vi "Autonomous Independent.vi"() -> ()   [LabVIEW 2014]
doc: "This VI is called when autonomous begins, and will automatically be terminated when autonomous ends. You can carry out timed or sensor driven robot movement independently without needing to return to the caller."
uses:
  <vilib>/Rock Robotics/WPI/RobotDrive/WPI_RobotDriveGetSetRefNum.vi
  <vilib>/Rock Robotics/Network Tables/SD Read Number.vi
  <vilib>/Utility/file.llb/Read From Spreadsheet File (DBL).vi
  <vilib>/Rock Robotics/WPI/RobotDrive/WPI_RobotDriveMecanumDrive_Cartesian.vi
  Robot Global Data.vi
panel:
  out "Autonomous Mode to run":T1(ring)
  in  "Ruin from Autonomous VI":bool
  out "Current State":string
  in  "Array":dbl[][](array[numeric])=[[0.0, 2.0], [3.0, 0.0], [0.0, 0.0], [0.0, 0.0]]
  # "[Drive]            [Rotate]             [Lift]                [ Strafe]              [Wait]"
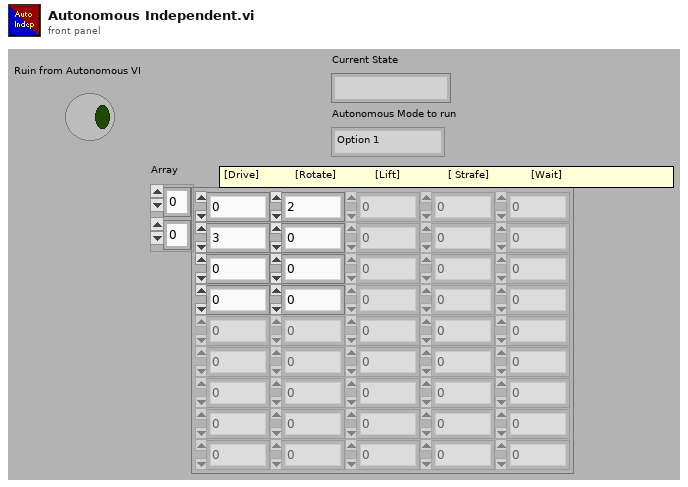
[diagram p1: front panel]
types:
  T1 = enum16{"Option 1", "Option 2", "Option 3", "Option 4", "Option 5", "Option 6"}
  T2 = typedef "WPI_RobotDriveDevRef.ctl" = cluster{"DevStatus":errorcluster, "Motors[]":T3[], "Square Inputs":bool, "Max Output":dbl}
  T3 = typedef "WPI_MotorControlDeviceRef.ctl" = cluster{"DeviceStatus":errorcluster, "Type":T4, "PWM":cluster{"Controller":T5, "PWM Channel":T6, "DeadBand":T7}, "CAN":cluster{"Device Number":u8, "Control Mode":T8, "Semaphore":T9, "Max Vout":dbl, "TalonSRX Control Mode":T10}, "Invert":bool, "TransformRef":T11, "InvTransformRef":T11}
  T4 = typedef "WPI_MotorControlType.ctl" = enum16{"PWM", "CAN", "CANTalonSRX"}
  T5 = typedef "FPGA_TypedefDigitalModule.ctl" = enum16{"Controller 1"}
  T6 = typedef "FPGA_DIOPWMChannel.ctl" = enum8{"PWM 0", "PWM 1", "PWM 2", "PWM 3", "PWM 4", "PWM 5", "PWM 6", "PWM 7", "PWM 8", "PWM 9", "PWM MXP 0", "PWM MXP 1", "PWM MXP 2", "PWM MXP 3", "PWM MXP 4", "PWM MXP 5", "PWM MXP 6", "PWM MXP 7", "PWM MXP 8", "PWM MXP 9", "Invalid"}
  T7 = typedef "WPI_PWMDeadband.ctl" = cluster{"Name":string, "maxPositivePwm":i32, "minPositivePwm":i32, "centerPwm":i32, "maxNegativePwm":i32, "minNegativePwm":i32, "angularRange":u16}
  T8 = typedef "WPI_CANJaguar_ControlMode.ctl" = enum8{"Percent VBus", "Current", "Speed", "Position", "Voltage"}
  T9 = typedef "Semaphore RefNum" = refnum<k1>
  T10 = typedef "WPI_CANTalonSRX_APIControlMode.ctl" = enum8{"Percent VBus", "Speed", "Position", "Slave", "Unchanged / Invalid"}
  T11 = typedef "WPI_PWMTransform_ConPane.ctl" = refnum<vi>
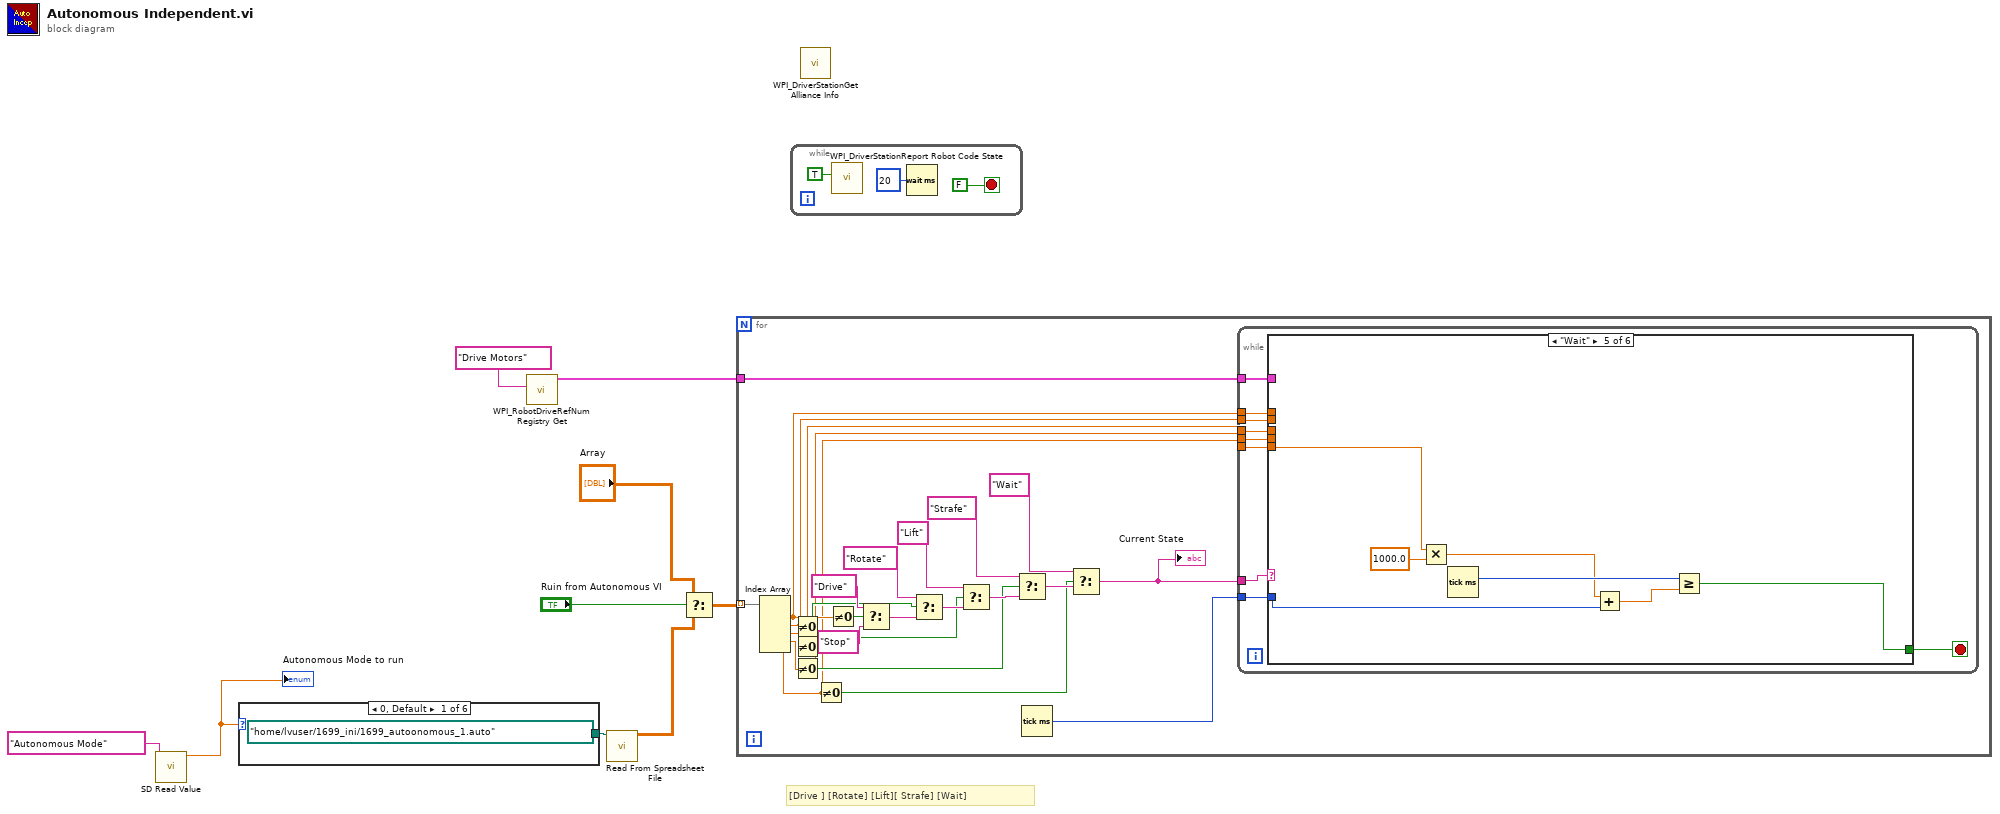
[diagram p0: block diagram]
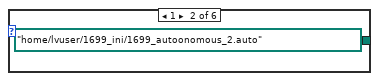
[diagram p2: hidden frame]
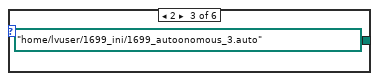
[diagram p3: hidden frame]
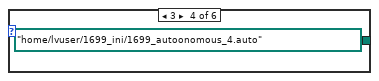
[diagram p4: hidden frame]
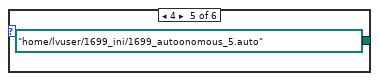
[diagram p5: hidden frame]
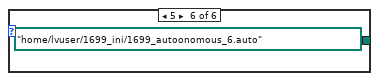
[diagram p6: hidden frame]
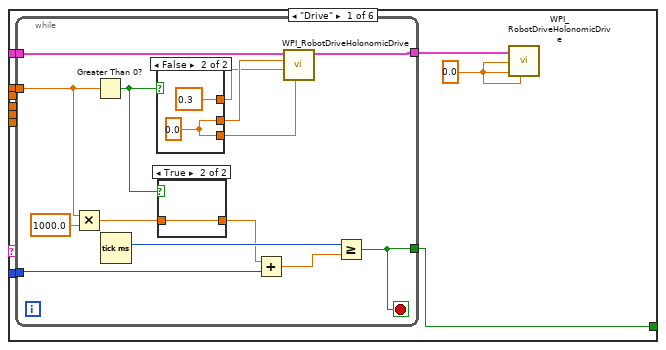
[diagram p7: hidden frame]
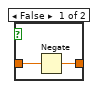
[diagram p8: hidden frame]
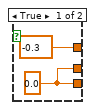
[diagram p9: hidden frame]
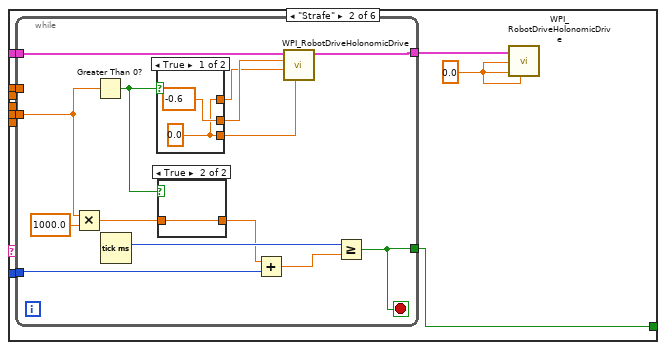
[diagram p10: hidden frame]
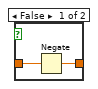
[diagram p11: hidden frame]
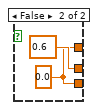
[diagram p12: hidden frame]
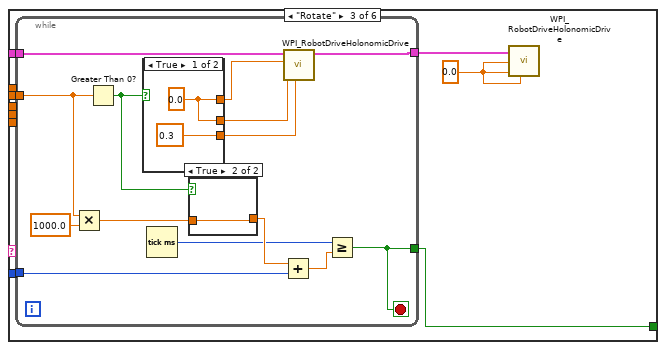
[diagram p13: hidden frame]
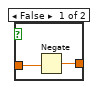
[diagram p14: hidden frame]
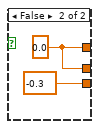
[diagram p15: hidden frame]
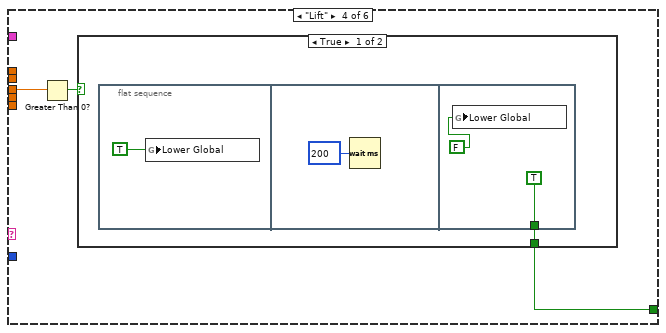
[diagram p16: hidden frame]
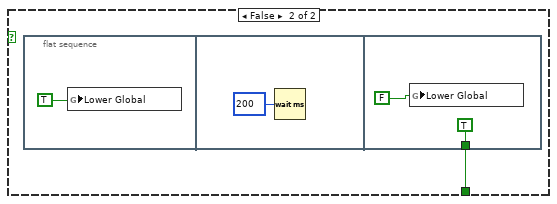
[diagram p17: hidden frame]
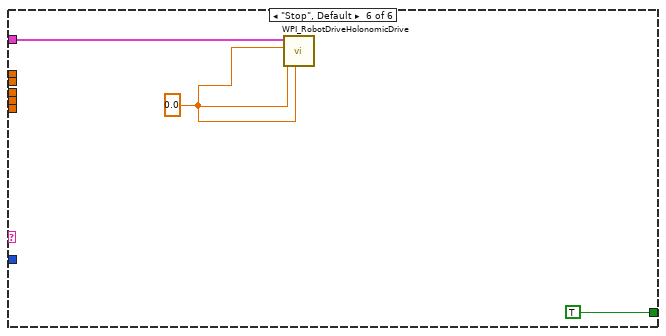
[diagram p18: hidden frame]
diagram:
  # "[Drive ] [Rotate] [Lift][ Strafe] [Wait]"
  n1 = call-poly <vilib>:"SD Read Value.vi"("Name"="Autonomous Mode") -> ("Numeric"=w2:dbl)  [unwired: 8 in, 2 out]
  "Autonomous Mode to run" <- w2
  n2 = case shown="0, Default" w2 {
    tunnel: [path "/home/lvuser/1699_ini/1699_autoonomous_1.auto" ("configuration file path") path "/home/lvuser/1699_ini/1699_autoonomous_2.auto" ("configuration file path") path "/home/lvuser/1699_ini/1699_autoonomous_3.auto" ("configuration file path") path "/home/lvuser/1699_ini/1699_autoonomous_4.auto" ("configuration file path") path "/home/lvuser/1699_ini/1699_autoonomous_5.auto" ("configuration file path") path "/home/lvuser/1699_ini/1699_autoonomous_6.auto" ("configuration file path")] -> w5
    frame 0, Default {
    }
    frame 1 {
    }
    frame 2 {
    }
    frame 3 {
    }
    frame 4 {
    }
    frame 5 {
    }
  }
  n3 = call <vilib>:"WPI_RobotDriveRefNum Registry Get.vi"("refnum name"="Drive Motors") -> ("RobotDriveDevRef"=w9:T2)  [unwired: 9 in, 1 out]
  n4 = call-poly <vilib>:"Read From Spreadsheet File.vi"("file path (dialog if empty)"=w5) -> ("all rows"=w4:dbl[][])  [unwired: 6 in, 4 out]
  n5 = Select(t="Array", s="Ruin from Autonomous VI", f=w4) -> (s? t:f=w7:dbl[][])
  n6 = for {
    tunnel: w9 -> [w27]
    tunnel: w7 -> [w21] mode=indexing
    n7 = Index Array(array=w21) -> (element #1=w26:dbl, element #2=w24:dbl, element #3=w23:dbl, element #4=w22:dbl, element #5=w16:dbl)  [unwired: 5 in]
    n8 = Not Equal To 0?(x=w24) -> (x != 0?=w30:bool)
    n9 = Not Equal To 0?(x=w23) -> (x != 0?=w29:bool)
    n10 = Not Equal To 0?(x=w22) -> (x != 0?=w28:bool)
    n11 = Not Equal To 0?(x=w16) -> (x != 0?=w19:bool)
    n12 = Not Equal To 0?(x=w26) -> (x != 0?=w39:bool)
    n13 = Select(t="Drive", s=w39, f="Stop") -> (s? t:f=w36:string)
    n14 = Select(t="Rotate", s=w30, f=w36) -> (s? t:f=w34:string)
    n15 = Select(t="Lift", s=w29, f=w34) -> (s? t:f=w32:string)
    n16 = Select(t="Strafe", s=w28, f=w32) -> (s? t:f=w20:string)
    n17 = Tick Count (ms)() -> (millisecond timer value=w25:u32)
    n18 = Select(t="Wait", s=w19, f=w20) -> (s? t:f=w17:string)
    "Current State" <- w17
    n19 = while {
      tunnel: w17 -> [w48]
      tunnel: w27 -> [w47]
      tunnel: w26 -> [w46]
      tunnel: w25 -> [w45]
      tunnel: w24 -> [w44]
      tunnel: w23 -> [w43]
      tunnel: w22 -> [w42]
      tunnel: w16 -> [w40]
      stop <- w41 stop-if-true
      n20 = case shown="\"Wait\"" w48 {
        tunnel: w47 -> [w53 w81 w108 _ _ w153]
        tunnel: w46 -> [w51 w79 _ _ _ _]
        tunnel: w45 -> [w50 w78 w106 _ w146 _]
        tunnel: w44 -> [_ _ w105 _ _ _]
        tunnel: w43 -> [_ _ _ w133 _ _]
        tunnel: w42 -> [_ w76 _ _ _ _]
        tunnel: [w49 w77 w104 w131 w145 TRUE] -> w41
        tunnel: w40 -> [_ _ _ _ w144 _]
        frame "Drive" {
          w54 = 0.0 ("X")
          n21 = while {
            tunnel: w53 -> [w67]
            tunnel: [w66] -> w52
            tunnel: w51 -> [w65]
            tunnel: w50 -> [w62]
            tunnel: [w60] -> w49
            stop <- w60 stop-if-true
            n22 = Multiply(x=w65, y=1000.0) -> (x*y=w58:dbl)
            n23 = Greater Than 0?(x=w65) -> (x > 0?=w59:bool)
            n24 = Tick Count (ms)() -> (millisecond timer value=w63:u32)
            n25 = case shown="False" w59 {
              tunnel: [-0.3 ("X") 0.3 ("X")] -> w55
              tunnel: [w72 w74] -> w56
              tunnel: [w72 w74] -> w68
              frame True {
                w72 = 0.0 ("Rotation")
              }
              frame False {
                w74 = 0.0 ("Rotation")
              }
            }
            n26 = case shown="True" w59 {
              tunnel: w58 -> [w69 w71]
              tunnel: [w70 w71] -> w57
              frame False {
                n27 = Negate(x=w69) -> (-x=w70:dbl)
              }
              frame True {
              }
            }
            n28 = Add(x=w57, y=w62) -> (x+y=w61:dbl)
            n29 = call-poly <vilib>:"WPI_RobotDriveHolonomicDrive.vi"("Rotation"=w68, "Y"=w55, "X"=w56, "RobotDriveDevRef"=w67) -> ("RobotDriveDevRef"=w66:T2)  [unwired: 5 in, 2 out]
            n30 = Greater Or Equal?(x=w63, y=w61) -> (x >= y?=w60:bool)
          }
          n31 = call-poly <vilib>:"WPI_RobotDriveHolonomicDrive.vi"("Rotation"=w54, "Y"=w54, "X"=w54, "RobotDriveDevRef"=w52) -> ()  [unwired: 5 in, 3 out]
        }
        frame "Strafe" {
          w82 = 0.0 ("X")
          n32 = while {
            tunnel: w81 -> [w95]
            tunnel: [w94] -> w80
            tunnel: w79 -> [_]
            tunnel: w78 -> [w91]
            tunnel: [w89] -> w77
            tunnel: w76 -> [w83]
            stop <- w89 stop-if-true
            n33 = Multiply(x=w83, y=1000.0) -> (x*y=w87:dbl)
            n34 = Greater Than 0?(x=w83) -> (x > 0?=w88:bool)
            n35 = Tick Count (ms)() -> (millisecond timer value=w92:u32)
            n36 = case shown="True" w88 {
              tunnel: [w100 w102] -> w84
              tunnel: [-0.6 ("X") 0.6 ("X")] -> w85
              tunnel: [w100 w102] -> w96
              frame True {
                w100 = 0.0 ("Rotation")
              }
              frame False {
                w102 = 0.0 ("Rotation")
              }
            }
            n37 = case shown="True" w88 {
              tunnel: w87 -> [w97 w99]
              tunnel: [w98 w99] -> w86
              frame False {
                n38 = Negate(x=w97) -> (-x=w98:dbl)
              }
              frame True {
              }
            }
            n39 = Add(x=w86, y=w91) -> (x+y=w90:dbl)
            n40 = call-poly <vilib>:"WPI_RobotDriveHolonomicDrive.vi"("Rotation"=w96, "Y"=w84, "X"=w85, "RobotDriveDevRef"=w95) -> ("RobotDriveDevRef"=w94:T2)  [unwired: 5 in, 2 out]
            n41 = Greater Or Equal?(x=w92, y=w90) -> (x >= y?=w89:bool)
          }
          n42 = call-poly <vilib>:"WPI_RobotDriveHolonomicDrive.vi"("Rotation"=w82, "Y"=w82, "X"=w82, "RobotDriveDevRef"=w80) -> ()  [unwired: 5 in, 3 out]
        }
        frame "Rotate" {
          w109 = 0.0 ("X")
          n43 = while {
            tunnel: w108 -> [w121]
            tunnel: [w120] -> w107
            tunnel: w106 -> [w118]
            tunnel: w105 -> [w116]
            tunnel: [w115] -> w104
            stop <- w115 stop-if-true
            n44 = Multiply(x=w116, y=1000.0) -> (x*y=w113:dbl)
            n45 = Greater Than 0?(x=w116) -> (x > 0?=w114:bool)
            n46 = case shown="True" w114 {
              tunnel: [w127 w129] -> w117
              tunnel: [w127 w129] -> w123
              tunnel: [0.3 ("Rotation") -0.3 ("Rotation")] -> w122
              frame True {
                w127 = 0.0 ("X")
              }
              frame False {
                w129 = 0.0 ("X")
              }
            }
            n47 = Tick Count (ms)() -> (millisecond timer value=w111:u32)
            n48 = case shown="True" w114 {
              tunnel: [w125 w126] -> w112
              tunnel: w113 -> [w124 w126]
              frame False {
                n49 = Negate(x=w124) -> (-x=w125:dbl)
              }
              frame True {
              }
            }
            n50 = Add(x=w112, y=w118) -> (x+y=w110:dbl)
            n51 = call-poly <vilib>:"WPI_RobotDriveHolonomicDrive.vi"("Rotation"=w122, "Y"=w123, "X"=w117, "RobotDriveDevRef"=w121) -> ("RobotDriveDevRef"=w120:T2)  [unwired: 5 in, 2 out]
            n52 = Greater Or Equal?(x=w111, y=w110) -> (x >= y?=w115:bool)
          }
          n53 = call-poly <vilib>:"WPI_RobotDriveHolonomicDrive.vi"("Rotation"=w109, "Y"=w109, "X"=w109, "RobotDriveDevRef"=w107) -> ()  [unwired: 5 in, 3 out]
        }
        frame "Lift" {
          n54 = Greater Than 0?(x=w133) -> (x > 0?=w132:bool)
          n55 = case shown="True" w132 {
            tunnel: [w134 w139] -> w131
            frame True {
              n56 = flat-sequence {
                tunnel: [TRUE] -> w134
                frame #0 {
                  n57 = global write "Robot Global Data.vi" "Lower Global"(TRUE ("Lift Global")) -> ()
                }
                frame #1 {
                  n58 = Wait (ms)(milliseconds to wait=u32 200) -> ()  [unwired: 1 out]
                }
                frame #2 {
                  n59 = global write "Robot Global Data.vi" "Lower Global"(FALSE ("Lift Global")) -> ()
                }
              }
            }
            frame False {
              n60 = flat-sequence {
                tunnel: [TRUE] -> w139
                frame #0 {
                  n61 = global write "Robot Global Data.vi" "Lower Global"(TRUE ("Lift Global")) -> ()
                }
                frame #1 {
                  n62 = Wait (ms)(milliseconds to wait=u32 200) -> ()  [unwired: 1 out]
                }
                frame #2 {
                  n63 = global write "Robot Global Data.vi" "Lower Global"(FALSE ("Lift Global")) -> ()
                }
              }
            }
          }
        }
        frame "Wait" {
          n64 = Multiply(x=w144, y=1000.0) -> (x*y=w147:dbl)
          n65 = Tick Count (ms)() -> (millisecond timer value=w149:u32)
          n66 = Add(x=w147, y=w146) -> (x+y=w150:dbl)
          n67 = Greater Or Equal?(x=w149, y=w150) -> (x >= y?=w145:bool)
        }
        frame "Stop", Default {
          w152 = 0.0 ("Rotation")
          n68 = call-poly <vilib>:"WPI_RobotDriveHolonomicDrive.vi"("Rotation"=w152, "Y"=w152, "X"=w152, "RobotDriveDevRef"=w153) -> ()  [unwired: 5 in, 3 out]
        }
      }
    }
  }
  n69 = while {
    stop <- FALSE stop-if-true
    n70 = call <vilib>:"WPI_DriverStationReport Robot Code State.vi"("Autonomous"=TRUE) -> ()  [unwired: 10 in, 1 out]
    n71 = Wait (ms)(milliseconds to wait=u32 20) -> ()  [unwired: 1 out]
  }
  n72 = call <vilib>:"WPI_DriverStationGet Alliance Info.vi"() -> ()  [unwired: 12 out]
